vi "Combined Status Monitor and Transient Capture (Array of Units Under Test).vi"() -> ()   [LabVIEW 2017]
uses:
  Communications/Communications Library.lvlib
panel:
  in  "Previous Button":bool
  in  "Next Button":bool
  out "Currently Selected Unit Under Test":string
  out "Array of Units Under Test":T1(array[cluster])
  in  "Graph":bool
  in  "Arm":bool
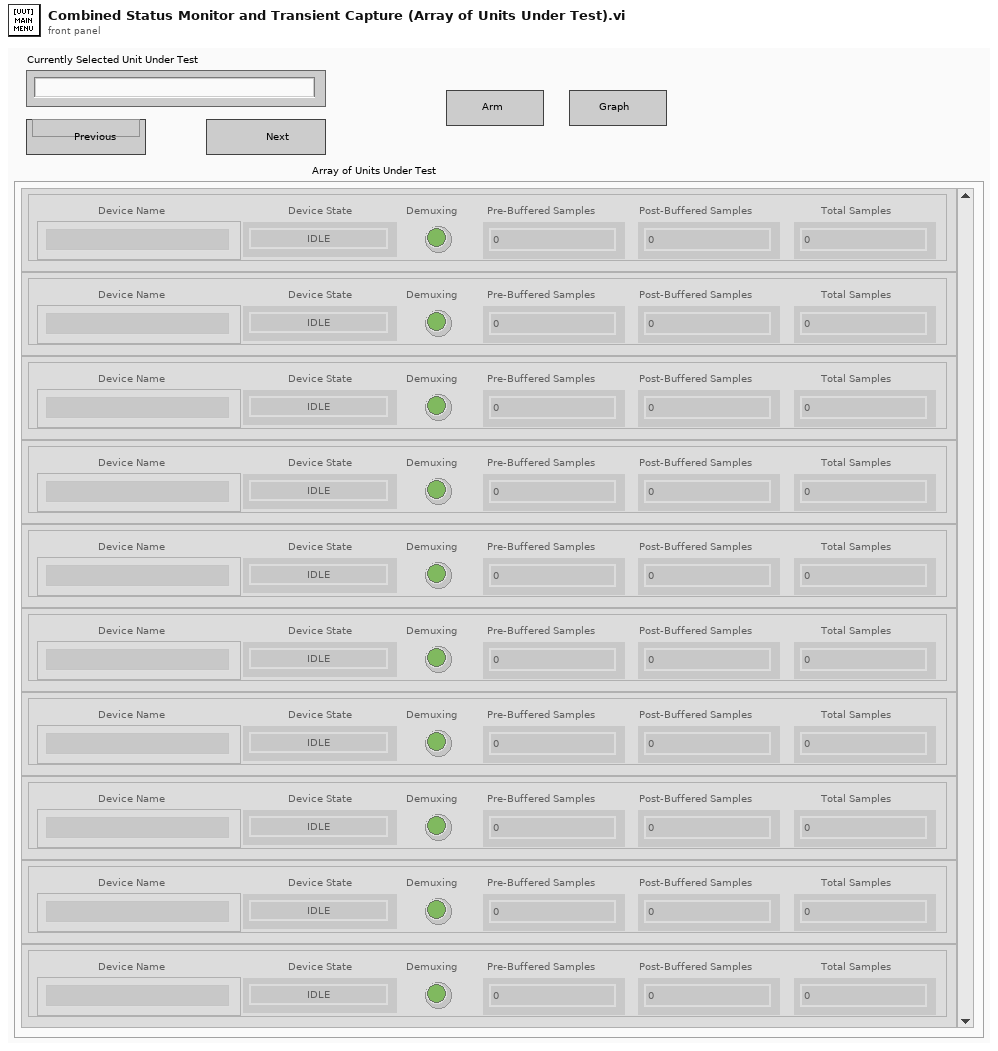
[diagram p1: front panel]
types:
  T1 = cluster{"Device State":enum16{"IDLE", "ARM", "RUN_PRE-TRIGGER", "RUN_POST-TRIGGER", "POST_PROCESS", "CLEANUP"}, "Pre-Buffered Samples":i32, "Post-Buffered Samples":i32, "Total Samples":i32, "Demuxing":bool, "Device Name":string}[]
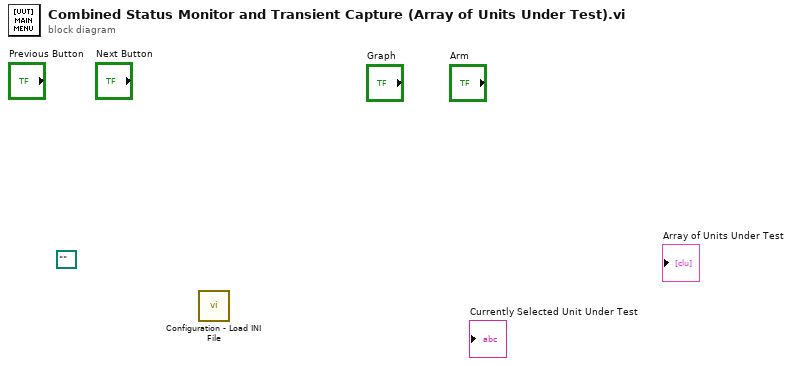
[diagram p0: block diagram]
diagram:
  (unwired) path "" ("configuration file path")
  n1 = call "Configuration - Load INI File.vi"() -> ("configuration file path"=w1:path)  [unwired: 9 in, 2 out]
